vi "Marshall (binary).vi"(8 "error in (no error)":errorcluster, 10 "Variant":variant, 11 "Serializer in":refnum<class "Serializer.lvclass">) -> (0 "error out":errorcluster, 2 "Bytes":u8[](array[numeric]) format="%08b", 3 "Serializer out":refnum<class "Serializer.lvclass">)   [LabVIEW 2013, in "OpenSerializer.lvlib" / "Serializer.lvclass"]
uses:
  Serializer.lvclass
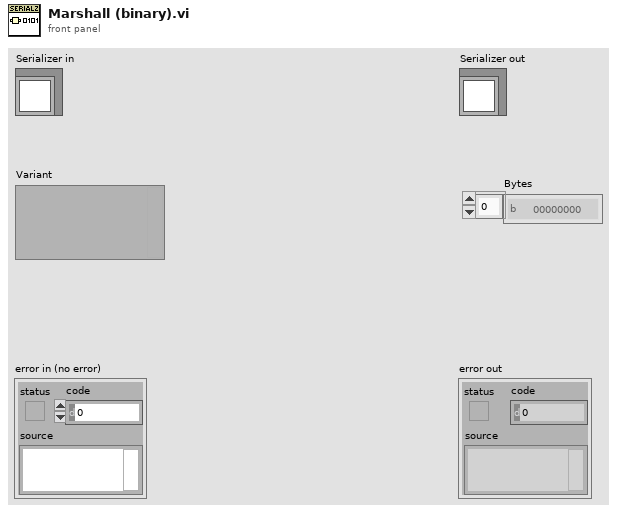
[diagram p1: front panel]
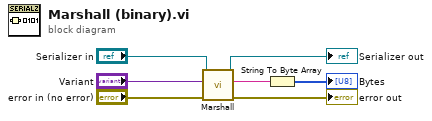
[diagram p0: block diagram]
diagram:
  n1 = call "Marshall.vi"("error in (no error)"="error in (no error)", "Variant"="Variant", "Serializer in"="Serializer in") -> ("error out"=→"error out":errorcluster, "String"=w4:string, "Serializer out"=→"Serializer out":refnum<class "Serializer.lvclass">)  [unwired: 6 in]
  n2 = String To Byte Array(string=w4) -> (unsigned byte array=→"Bytes":u8[])
